vi "LVClass_WavefrontCorrector Assert User Prefs and Move to Relative Position.vi"(0 "WavefrontCorrector in":refnum<class "WavefrontCorrector.lvclass">, 2 "Check position before move":bool, 5 "Wavefront Corrector State":T1[](array[typedef]), 7 "Sleep after command apply (ms)":i32, 9 "Relative Positions":T2, 11 "error in (no error)":errorcluster) -> (4 "WavefrontCorrector out":refnum<class "WavefrontCorrector.lvclass">, 15 "error out":errorcluster)   [LabVIEW 2020, in "WavefrontCorrector.lvclass"]
uses:
  WavefrontCorrector.lvclass
  Wavefront Corrector Position.ctl
  Wavefront Corrector states - ONE.ctl
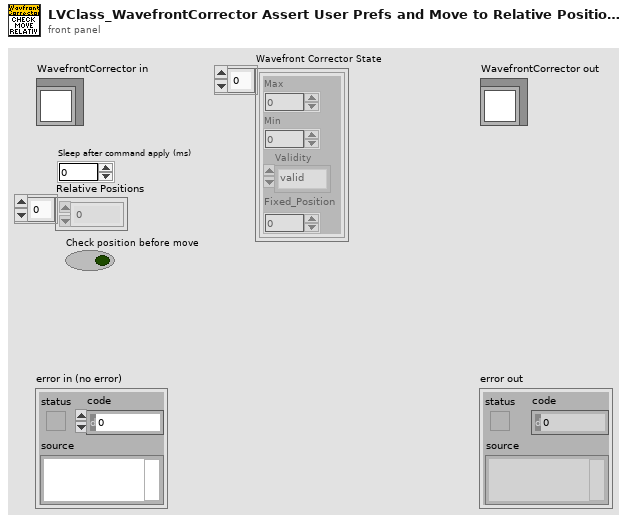
[diagram p1: front panel]
types:
  T1 = typedef "Wavefront Corrector states - ONE.ctl" = cluster{"Max":sgl, "Min":sgl, "Validity":enum16{"valid", "fixed", "invalid"}, "Fixed_Position":sgl}
  T2 = typedef "Wavefront Corrector Position.ctl" = sgl[]
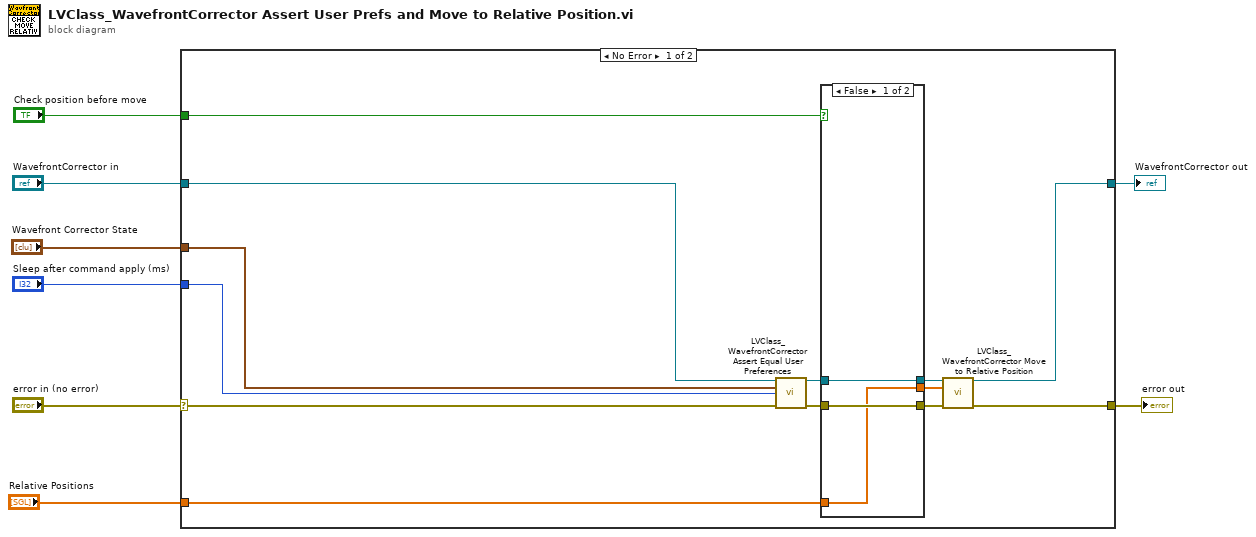
[diagram p0: block diagram]
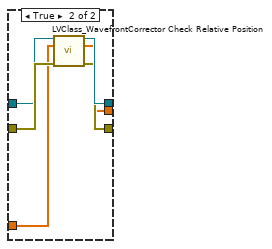
[diagram p2: hidden frame]
diagram:
  n1 = case shown="No Error" "error in (no error)" {
    selector: "error in (no error)" -> [w16 w32]
    tunnel: [w18 w32] -> w5
    tunnel: [w20 w31] -> w6
    tunnel: "WavefrontCorrector in" -> [w12 w31]
    tunnel: "Check position before move" -> [w13 _]
    tunnel: "Sleep after command apply (ms)" -> [w9 _]
    tunnel: "Relative Positions" -> [w11 _]
    tunnel: "Wavefront Corrector State" -> [w10 _]
    frame No Error {
      n2 = call "LVClass_WavefrontCorrector Assert Equal User Preferences.vi"("WavefrontCorrector in"=w12, "Wavefront Corrector State"=w10, "Sleep after command apply (ms)"=w9, "error in (no error)"=w16) -> ("WavefrontCorrector out"=w14:refnum<class "WavefrontCorrector.lvclass">, "error out"=w15:errorcluster)  [unwired: 10 in]
      n3 = case shown="False" w13 {
        tunnel: [w24 w30] -> w21
        tunnel: [w23 w29] -> w19
        tunnel: [w22 w28] -> w17
        tunnel: w15 -> [w23 w27]
        tunnel: w14 -> [w24 w26]
        tunnel: w11 -> [w22 w25]
        frame False {
        }
        frame True {
          n4 = call "LVClass_WavefrontCorrector Check Relative Position.vi"("WavefrontCorrector in"=w26, "Relative Positions"=w25, "error in (no error)"=w27) -> ("WavefrontCorrector out"=w30:refnum<class "WavefrontCorrector.lvclass">, "Relative Positions OUT"=w28:T2, "error out"=w29:errorcluster)  [unwired: 10 in]
        }
      }
      n5 = call "LVClass_WavefrontCorrector Move to Relative Position.vi"("WavefrontCorrector in"=w21, "Wavefront Relative Position"=w17, "error in (no error)"=w19) -> ("WavefrontCorrector out"=w20:refnum<class "WavefrontCorrector.lvclass">, "error out"=w18:errorcluster)  [unwired: 11 in]
    }
    frame Error {
    }
  }
  "error out" <- w5
  "WavefrontCorrector out" <- w6
